vi "OFDM-SIM信道.vi"(3 "数值":i32, 4 "采样率":dbl format="%#_13g", 5 "发射信号":cdb[](array[numeric])) -> (0 "信噪比":dbl format="%#_13g", 1 "接收信号2":cdb[](array[numeric]) format="%#_13g", 2 "接收信号":cluster{"t0":dbl, "dt":dbl, "Y":cdb[]})   [LabVIEW 2018]
uses:
  <vilib>/Analysis/baseanly.llb/Mean (DBL).vi
  <vilib>/Analysis/NI_AALBase.lvlib
panel:
  in  "初值":i32
  in  "步长":dbl=0.5 format="%#_13g"
  out "信号功率":dbl format="%#_13g"
  out "噪声功率":dbl format="%#_13g"
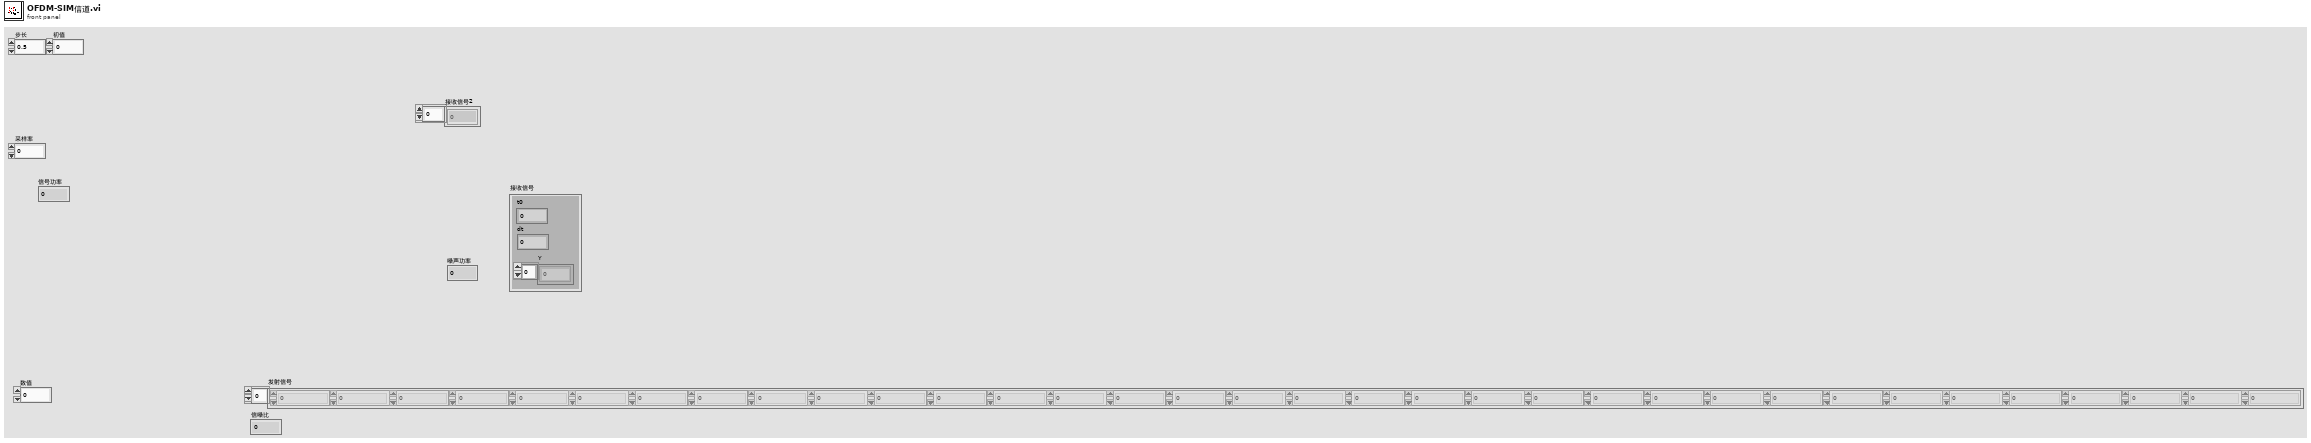
[diagram p1: front panel]
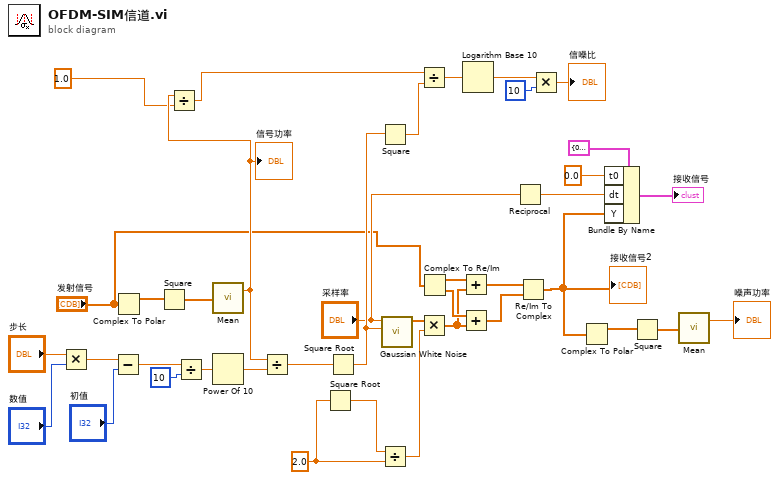
[diagram p0: block diagram]
diagram:
  w9 = 2.0
  n1 = Multiply(x="步长", y="数值") -> (x*y=w19:dbl)
  n2 = Subtract(x=w19, y="初值") -> (x-y=w21:dbl)
  n3 = Complex To Polar(r * e^(i*theta)="发射信号") -> (r=w35:dbl[])  [unwired: 1 out]
  n4 = Square(x=w35) -> (x^2=w14:dbl[])
  n5 = Divide(x=w21, y=10) -> (x/y=w25:dbl)
  n6 = call-poly <vilib>:"Mean.vi"("X"=w14) -> ("mean"=w5:dbl)  [unwired: 1 out]
  "信号功率" <- w5
  n7 = Divide(x=w5, y=1.0) -> (x/y=w4:dbl)
  n8 = Power Of 10(x=w25) -> (10^x=w24:dbl)
  n9 = Divide(x=w5, y=w24) -> (x/y=w23:dbl)
  n10 = Square Root(x=w9) -> (sqrt(x)=w10:dbl)
  n11 = Square Root(x=w23) -> (sqrt(x)=w22:dbl)
  n12 = Square(x=w22) -> (x^2=w27:dbl)
  n13 = Divide(x=w10, y=w9) -> (x/y=w8:dbl)
  n14 = call <vilib>:"Gaussian White Noise.vi"("standard deviation"=w22, "samples"="采样率") -> ("Gaussian noise pattern"=w7:dbl[])  [unwired: 8 in, 1 out]
  n15 = Divide(x=w4, y=w27) -> (x/y=w34:dbl)
  n16 = Multiply(x=w7, y=w8) -> (x*y=w6:dbl[])
  n17 = Complex To Re/Im(x + iy="发射信号") -> (x=w31:dbl[], y=w30:dbl[])
  n18 = Add(x=w31, y=w6) -> (x+y=w29:dbl[])
  n19 = Add(x=w30, y=w6) -> (x+y=w28:dbl[])
  n20 = Logarithm Base 10(1:w34) -> (0:w33:dbl)
  n21 = Reciprocal(x="采样率") -> (1/x=w38:dbl)
  n22 = Re/Im To Complex(1:w28, 2:w29) -> (0:w1:cdb[])
  "接收信号2" <- w1
  n23 = Multiply(x=w33, y=10) -> (x*y=→"信噪比":dbl)
  n24 = Complex To Polar(r * e^(i*theta)=w1) -> (r=w13:dbl[])  [unwired: 1 out]
  n25 = Bundle By Name(cluster=cluster{"t0":dbl, "dt":dbl, "Y":cdb[]} {"t0"=0.0, "dt"=1.0, "Y"=[]} ("IQ data (complex) in"), "t0"=0.0, "dt"=w38, "Y"=w1) -> (→"接收信号":cluster{"t0":dbl, "dt":dbl, "Y":cdb[]})
  n26 = Square(x=w13) -> (x^2=w12:dbl[])
  n27 = call-poly <vilib>:"Mean.vi"("X"=w12) -> ("mean"=→"噪声功率":dbl)  [unwired: 1 out]
